vi "Get DDG Step Mode.vi"(8 "error in (no error)":errorcluster, 11 "mode":u32) -> (0 "error out":errorcluster, 2 "function return":u32, 3 "mode out":u32)   [LabVIEW 2014, in "atmcd32d.lvlib"]
doc: "unsigned int WINAPI GetDDGStepMode(at_u32 * mode);"
uses:
  atmcd32d.lvlib
  atmcd32d.dll
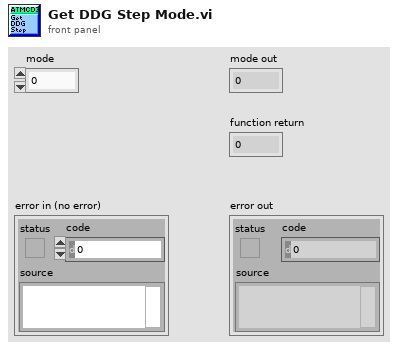
[diagram p1: front panel]
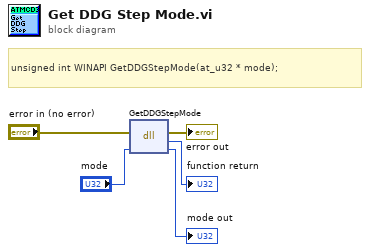
[diagram p0: block diagram]
diagram:
  # "unsigned int WINAPI GetDDGStepMode(at_u32 * mode);"
  n1 = dll-call lib="C:/Users/Bakir/Documents/Lambda2-Testing/lib/Andorlib/atmcd32d.*" fn="GetDDGStepMode"(error in="error in (no error)", "mode"="mode") -> (error out=→"error out":errorcluster, →"function return":u32, "mode"=→"mode out":u32)  [unwired: 2 in, 1 out]
